vi "Tx End.vi"(8 "error in (no error)":errorcluster, 11 "Performance in":refnum<class "Performance.lvclass">) -> (0 "error out":errorcluster, 3 "Performance out":refnum<class "Performance.lvclass">)   [LabVIEW 2017, in "DSF Core.lvlib" / "Performance.lvclass"]
uses:
  Performance.lvclass
  Performance.lvclass/Performance.ctl
  <vilib>/NI/Memory Manager/Classes/Pointer/Pointer.lvclass/Pointer.ctl
  <vilib>/NI/Memory Manager/Classes/Pointer/Write.vi
  <vilib>/NI/Memory Manager/Classes/Pointer/Write U32.vi
  <vilib>/NI/Memory Manager/Classes/Pointer/Write (No Check).vi
  <vilib>/NI/Memory Manager/Classes/Pointer/Write (No Check) U32.vi
  <vilib>/NI/Memory Manager/Classes/Pointer/Check Move.vi
  <vilib>/NI/Memory Manager/Classes/Pointer/Get Address.vi
  <vilib>/NI/Memory Manager/Classes/Pointer/Check Null Pointer.vi
  <vilib>/NI/Memory Manager/Classes/Pointer/Check Count.vi
  <vilib>/NI/Memory Manager/Classes/Pointer/Check Bounds (Power of 2).vi
  <vilib>/NI/Memory Manager/Classes/Pointer/Errors.vi
  <vilib>/NI/Memory Manager/Classes/Pointer/Null Pointer.vi
  <vilib>/NI/Memory Manager/Classes/Pointer/Is Null.vi
  <vilib>/NI/Memory Manager/Classes/Pointer/Get Size.vi
  <vilib>/NI/Memory Manager/Classes/Pointer/Out of Bounds.vi
  <vilib>/NI/Memory Manager/Classes/Pointer/Check Bounds.vi
  <vilib>/NI/Memory Manager/Classes/Pointer/Create Error.vi
  <vilib>/NI/Memory Manager/VIs/Source.Write.String.vi
  <vilib>/NI/Memory Manager/Classes/Pointer/Write Pointer Size.vi
  <vilib>/NI/Memory Manager/VIs/Source.Write.Scalar.Base10.vi
  <vilib>/NI/Memory Manager/VIs/Source.Write.Scalar.Base10 (U64).vi
  <vilib>/NI/Memory Manager/Classes/Pointer/Check Pointer Bounds.vi
  <vilib>/NI/Memory Manager/Classes/Pointer/Check Buffer Bounds.vi
  <vilib>/NI/Memory Manager/VIs/New Error Cluster Constant.vi
  <vilib>/NI/Memory Manager/VIs/New Error Cluster Constant (512B).vi
  <vilib>/NI/Memory Manager/VIs/Error Cluster.Set Status.vi
  <vilib>/NI/Memory Manager/VIs/Error Cluster.Set Code.vi
  <vilib>/NI/Memory Manager/VIs/Error Cluster.Set VI Source.vi
  <vilib>/NI/Memory Manager/Constants/Constants.vi
  <vilib>/NI/Memory Manager/Constants/Library Name.vi
  <vilib>/NI/Memory Manager/Classes/Pointer/Pointer Error Info.vi
  <vilib>/NI/Memory Manager/Constants/Pointer Class Name.vi
  <vilib>/NI/Memory Manager/Classes/Pointer/Buffer Underflow.vi
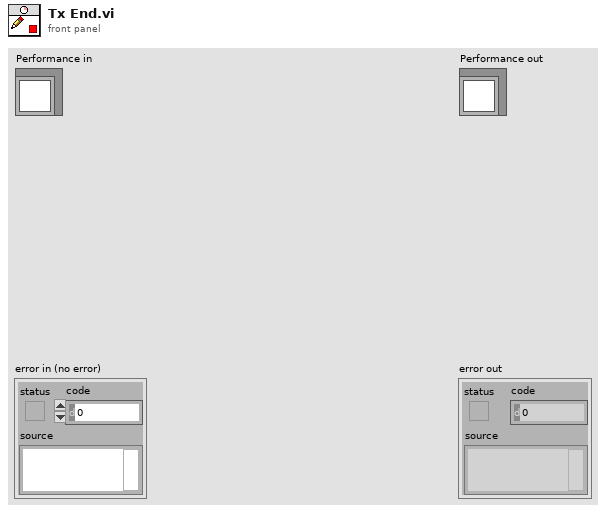
[diagram p1: front panel]
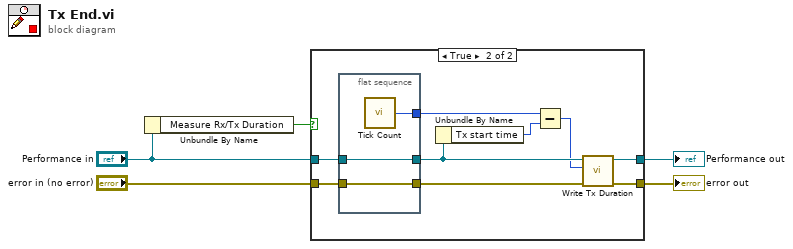
[diagram p0: block diagram]
diagram:
  n1 = Unbundle By Name("Performance in") -> ("Measure Rx/Tx Duration"=w1:bool)
  n2 = case shown="True" w1 {
    tunnel: [w6 w13] -> w5
    tunnel: "error in (no error)" -> [w6 w16]
    tunnel: [w7 w14] -> w3
    tunnel: "Performance in" -> [w7 w15]
    frame False {
    }
    frame True {
      n3 = flat-sequence {
        tunnel: w15 -> [w19]
        tunnel: w16 -> [w18]
        tunnel: [w19] -> w11
        tunnel: [w18] -> w12
        tunnel: [w17] -> w10
        frame #0 {
          n4 = call "Tick Count"() -> ("Tick Count(uSec)"=w17:u32)
        }
      }
      n5 = Unbundle By Name(w11) -> ("Tx start time"=w9:u32)
      n6 = Subtract(x=w10, y=w9) -> (x-y=w8:u32)
      n7 = call "Write Tx Duration.vi"("error in (no error)"=w12, "tx duration"=w8, "Framework Performance in"=w11) -> ("error out"=w13:errorcluster, "Framework Performance out"=w14:refnum<class "Performance.lvclass">)  [unwired: 7 in]
    }
  }
  "error out" <- w5
  "Performance out" <- w3
